vi "Application Example Advanced.vi"() -> ()   [LabVIEW 2015]
uses:
  <vilib>/Automotive Diagnostic Command Set/Diagnostic Protocols.llb/DTC Descriptor.ctl
  _SubVIs/DPID Periodic Rate.ctl
  _SubVIs/DPID Parameters.ctl
  <vilib>/Automotive Diagnostic Command Set/Diagnostic Protocols.llb/Diagnostic Trouble Code.ctl
  Engine/SubVIs/GMLAN/_SubVIs/DTCStatusMask.ctl
  <vilib>/Automotive Diagnostic Command Set/Diagnostic Transport.llb/Property ID.ctl
  <vilib>/xnet/xnet.llb/XNET Frame CAN.ctl
  <vilib>/xnet/xnet.llb/XNET Frame Type CAN.ctl
  _SubVIs/CAN Frame.ctl
  <vilib>/Automotive Diagnostic Command Set/Diagnostic Transport.llb/Transport Protocol Selector.ctl
  Engine/SubVIs/GMLAN/_SubVIs/ReadDataByPacketIdentifier_SubFunctions.ctl
  Engine/SubVIs/GMLAN/_SubVIs/DisableNormalCommunication_Parameter.ctl
  Engine/SubVIs/GMLAN/_SubVIs/ReadDiagnosticInformation_ByStatus.vi
  <vilib>/Utility/error.llb/Clear Errors.vi
  Engine/SubVIs/GMLAN/Utilities/GMLAN Service Broadcast.vi
  Engine/SubVIs/GMLAN/Utilities/Convert Raw Data to DTCs.vi
  <vilib>/xnet/xnet.llb/XNET Create Session (Frame Input Queued).vi
  <vilib>/Automotive Diagnostic Command Set/Diagnostic Transport.llb/Diagnostic Service.vi
  <vilib>/Automotive Diagnostic Command Set/Diagnostic Transport.llb/Apply Success Failure Error.vi
  <vilib>/Automotive Diagnostic Command Set/Diagnostic Transport.llb/Diag Globals.vi
  <vilib>/Automotive Diagnostic Command Set/Diagnostic Transport.llb/Diagnostic Service Send.vi
  <vilib>/Automotive Diagnostic Command Set/Diagnostic Transport.llb/Diagnostic Response Recv.vi
  <vilib>/Automotive Diagnostic Command Set/Diagnostic Transport.llb/Apply Diagnostic Error.vi
  <vilib>/xnet/xnet.llb/XNET Read (Frame CAN).vi
  <vilib>/Automotive Diagnostic Command Set/Diagnostic Protocols.llb/Convert to Phys.vi
  <vilib>/xnet/xnet.llb/XNET Database Close (Database).vi
  <vilib>/addons/Automotive Diagnostic Command Set/NI_Automotive Diagnostic Command Set.lvlib
  Engine/SubVIs/GMLAN/GMLAN.lvlib
panel:
  in  "Enable Comm":bool
  out "Success?":bool=TRUE
  in  "Read DID":bool
  in  "Read PIDs":bool
  in  "Stop DPIDs":bool
  in  "Start DPIDs":bool
  in  "DTC Reset":bool
  in  "Read DTCs":bool
  in  "Setup DPIDs":bool
  in  "Enable Comm":bool
  in  "Write CPID":bool
  in  "Disable Comm":bool
  in  "Tab Control":T1(tab)
  in  "HW select":u16(ring) items=["NI-XNET", "NI-CAN"]
  in  "CAN Interface":string(combo)="CAN1"
  in  "Baudrate":u32=500000
  in  "Receive ID":u32=2024 format="%.0x"
  in  "Transmit ID":u32=2016 format="%.0x"
  in  "UUDT Receive ID":u32=1512 format="%.0x"
  in  "DPIDs":T3(array[cluster])=[{"DPID ID"=239, "Speed"=enum."Medium", "PIDs"=[14]}, {"DPID ID"=253, "Speed"=enum."Fast", "PIDs"=[12]}] {"PIDs" format="%.0x"; "DPID ID" format="%.0x"}
  in  "DTC descriptor":T4={"DTC Byte Length"=2, "Status Byte Length"=1, "Add Data Byte Length"=1, "Byte Order"=enum."Motorola"}
  in  "DID ID":u8=153 format="%.0x"
  out "DID Data":u8[](array[numeric])=[32, 8, 18, 17]
  out "PID Data":u8[](array[numeric])=[128]
  in  "PID ID":u16=14 format="%.0x"
  in  "CPID ID":u8=29 format="%.0x"
  in  "CPIDControlBytes":u8[](array[numeric])=[0, 0, 0, 0, 0] format="%.0x"
  out "DPID":T5={"DPID ID"=253, "Speed"=enum."Fast", "PIDs"=[12]}
  out "timestamp":timestamp=timestamp(3432175878.295675 s since 1904-01-01)
  out "payload":u8[](array[numeric])
  out "EndofDTCReport":bool=TRUE
  out "DTCs":T6[](array[typedef])
  in  "status mask":T7={"DTC supported by calibration"=FALSE, "current DTC"=TRUE, "test not passed since DTC cleared"=FALSE, "test failed since DTC cleared"=FALSE, "history DTC"=FALSE, "test not passed since current power up"=FALSE, "current DTC since power up"=FALSE, "warning indicator requested state"=FALSE}
  out "error IO":errorcluster
  in  "stop":bool
  out "stopped?":bool=TRUE
  # "$90 - VehicleIdentificationNumber (VIN)\n$92\t- System Supplier ID\n$97\t- SystemNameOrEngineType"
  # "$C - Engine Speed\n$E\t- Spark Advance"
  # "x10 CDAR\nx1D PHSR"
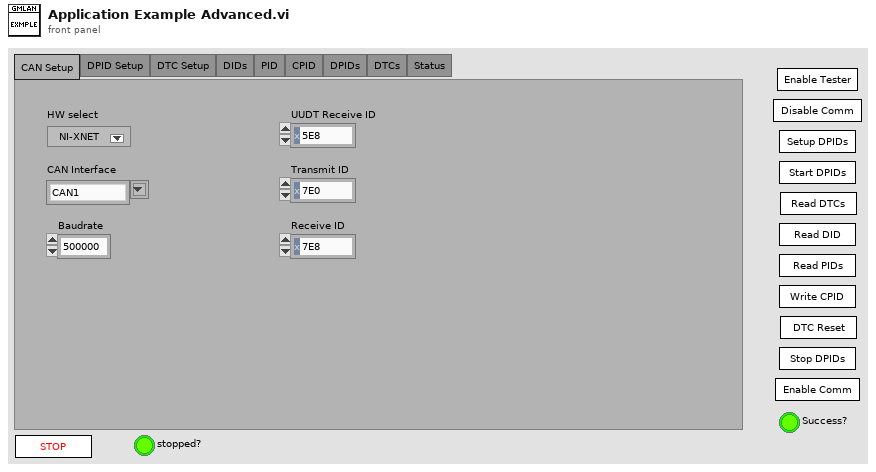
[diagram p1: front panel]
types:
  T1 = enum32{"CAN Setup", "DPID Setup", "DTC Setup", "DIDs", "PID", "CPID", "DPIDs", "DTCs", "Status"}
  T2 = typedef "DPID Periodic Rate.ctl" = enum16{"Slow", "Medium", "Fast"}
  T3 = cluster{"DPID ID":u8, "Speed":T2, "PIDs":u16[]}[]
  T4 = typedef "DTC Descriptor.ctl" = cluster{"DTC Byte Length":i32, "Status Byte Length":i32, "Add Data Byte Length":i32, "Byte Order":enum16{"Motorola", "Intel"}}
  T5 = typedef "DPID Parameters.ctl" = cluster{"DPID ID":u8, "Speed":T2, "PIDs":u16[]}
  T6 = typedef "Diagnostic Trouble Code.ctl" = cluster{"DTC":u32, "Status":u32, "Add Data":u32}
  T7 = typedef "GMLAN.lvlib/DTCStatusMask.ctl" = cluster{"DTC supported by calibration":bool, "current DTC":bool, "test not passed since DTC cleared":bool, "test failed since DTC cleared":bool, "history DTC":bool, "test not passed since current power up":bool, "current DTC since power up":bool, "warning indicator requested state":bool}
  T8 = typedef "CAN Frame.ctl" = cluster{"Frame name":string, "Identifier":u32, "Payload Length":u32, "Timing Type":u32, "Transmit Time":dbl, "Extended Identifier?":bool, "Comment":string}
  T9 = typedef "XNET Frame CAN.ctl" = cluster{"timestamp":timestamp, "payload":u8[], "identifier":u32, "type":T10, "extended?":bool, "echo?":bool}
  T10 = typedef "XNET Frame Type CAN.ctl" = u8
  T11 = typedef "NI_Automotive Diagnostic Command Set.lvlib/Property ID.ctl" = enum16{"Timeout Diag Command", "Timeout FC (Bs)", "Timeout CF (Cr)", "Receive Block Size (BS)", "Wait Time CF (STmin)", "Max Wait Frames (N_WFTmax)", "Wait Frames to Send (N_WAIT)", "Time between Waits (T_W)", "Fill CAN Frames", "Fill Byte", "Invalid Response as Error", "Max RspPending Count", "VWTP Command Timeout", "STmin", "P2min", "Termination"}
  T12 = typedef "NI_Automotive Diagnostic Command Set.lvlib/Transport Protocol Selector.ctl" = enum16{"ISO TP - Normal Mode", "ISO TP - Mixed Mode", "VW TP 2.0", "Diagnostics on IP", "ISO TP LIN"}
  T13 = typedef "NI_Automotive Diagnostic Command Set.lvlib/Diag Reference.ctl" = cluster{"Diag CAN Handle":u32, "Transport Protocol":T12, "Receive Address Extension":u8, "Transmit Address Extension":u8, "Receive CAN Id":u32, "Transmit CAN Id":u32, "Diag CAN Queue":refnum<queue>, "Log Frames ?":bool, "My TP Address":u8, "Other TP Address":u8, "T1":u16, "T2":u16, "T3":u16, "T4":u16, "Tx SN":u8, "Block Size":u8, "Rx SN":u8, "VW TP Initialized?":bool, "Tx block no":u8, "baud rate":u32, "Interface":string, "Channel Diag CAN Handle":u32, "UDP Connection ID":refnum<k16>, "TCP Connection ID":refnum<k5>, "Target IP Addr":u32, "Source Address":u16, "Target Address":u16, "Send Header NACK?":bool, "DLL Handle":u32, "NAD":u8, "Time Stamp read first":dbl, "Time Stamp read last":dbl, "Time Stamp write first":dbl, "Time Stamp write last":dbl, "Time Stamp write":dbl, "Time Stamp read":dbl}
  T14 = enum8{"Idle", "Read DID", "Read DTCs", "Reset DTCs", "Setup DPIDs", "Start DPIDs", "Stop DPIDs", "Read PID", "Write CPID", "DisableCommunication", "EnableCommunication", "Stop"}
  T15 = typedef "GMLAN.lvlib/ReadDataByPacketIdentifier_SubFunctions.ctl" = enum8{"stopSending", "sendOneResponse", "scheduleAtSlowRate", "scheduleAtMediumRate", "scheduleAtFastRate"}
  T16 = typedef "GMLAN.lvlib/DisableNormalCommunication_Parameter.ctl" = enum8{"SpecificECU", "EntireNetwork"}
  T17 = typedef "Filtered DPID IDs.ctl" = cluster{"Slow":u8[], "Medium":u8[], "Fast":u8[]}
  T18 = typedef "NI_Automotive Diagnostic Command Set.lvlib/Diag CAN Frame Log.ctl" = cluster{"Timestamp":dbl, "ArbitrationId":u32, "IsRemote":u8, "DataLength":u8, "Data":u8[]}
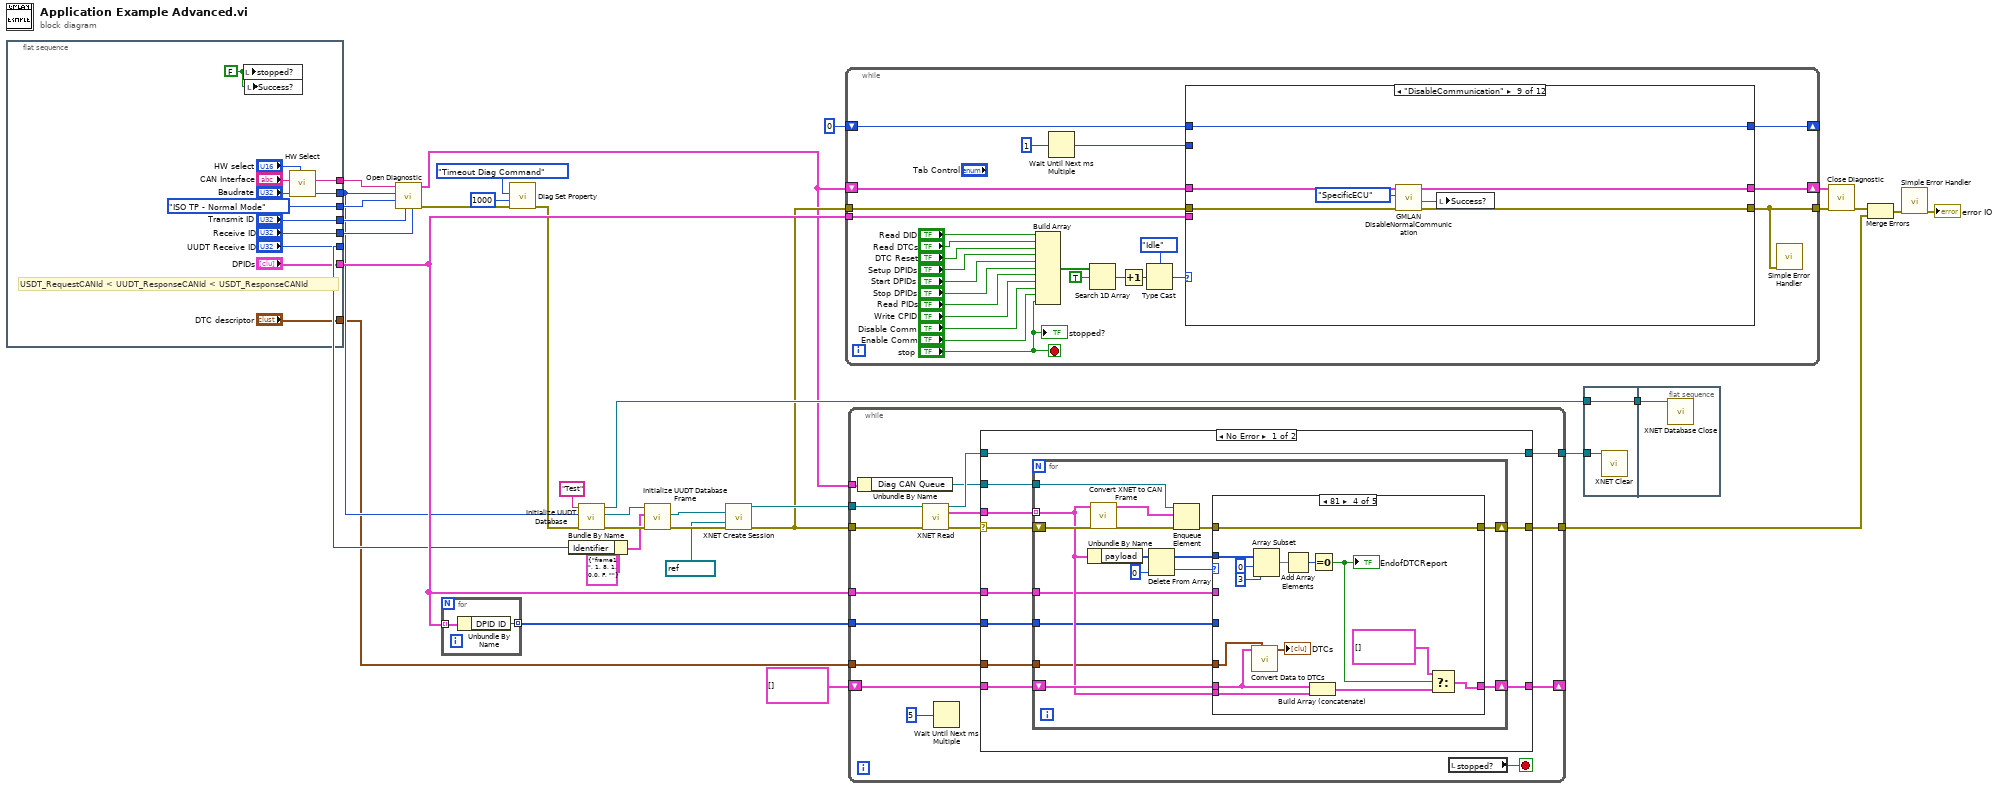
[diagram p0: block diagram]
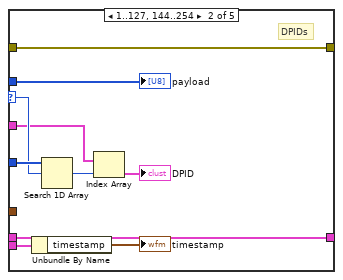
[diagram p3: hidden frame]
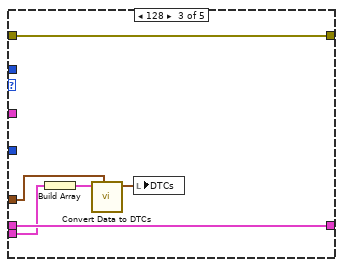
[diagram p4: hidden frame]
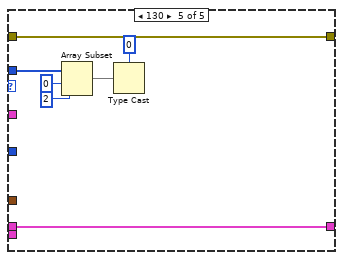
[diagram p5: hidden frame]
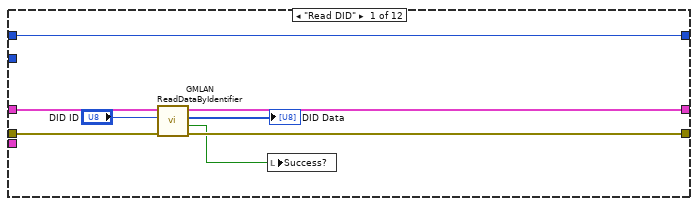
[diagram p7: hidden frame]
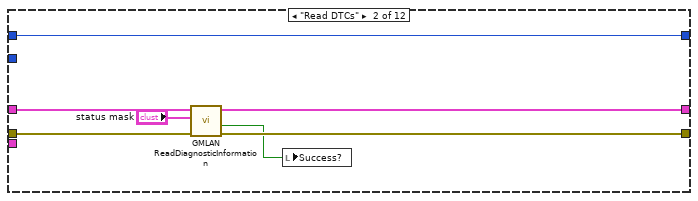
[diagram p8: hidden frame]
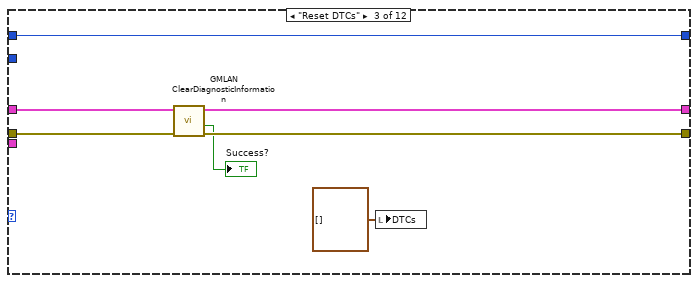
[diagram p9: hidden frame]
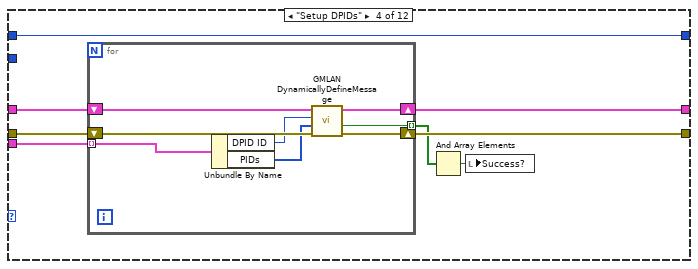
[diagram p10: hidden frame]
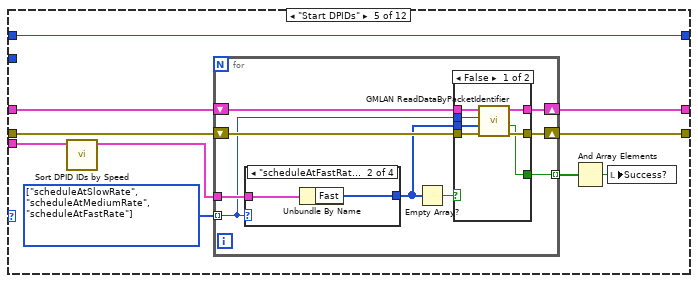
[diagram p11: hidden frame]
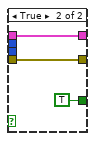
[diagram p12: hidden frame]
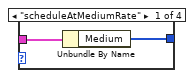
[diagram p13: hidden frame]
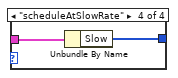
[diagram p15: hidden frame]
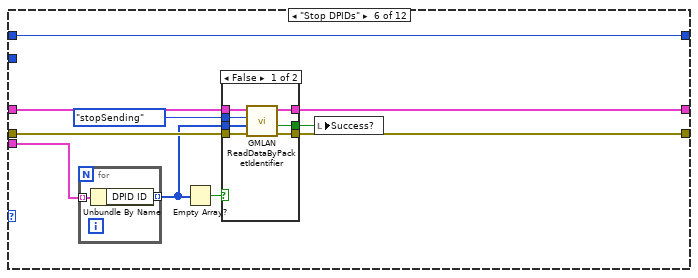
[diagram p16: hidden frame]
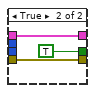
[diagram p17: hidden frame]
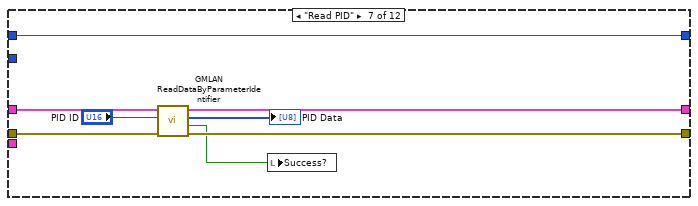
[diagram p18: hidden frame]
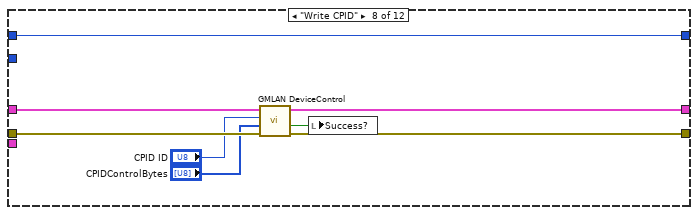
[diagram p19: hidden frame]
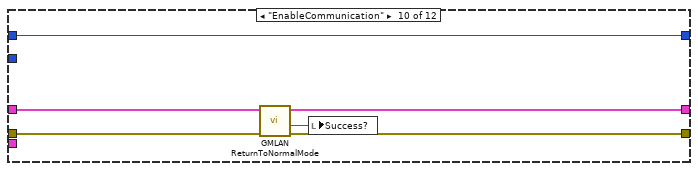
[diagram p20: hidden frame]
diagram:
  n1 = flat-sequence {
    tunnel: [w46] -> w33
    tunnel: ["Baudrate"] -> w2
    tunnel: [Transport_Protocol_Selector."ISO TP - Normal Mode" ("Transport Protocol")] -> w32
    tunnel: ["Transmit ID"] -> w31
    tunnel: ["Receive ID"] -> w30
    tunnel: ["UUDT Receive ID"] -> w11
    tunnel: ["DTC descriptor"] -> w1
    tunnel: ["DPIDs"] -> w20
    frame #0 {
      w36 = FALSE ("stopped?")
      # "USDT_RequestCANId < UUDT_ResponseCANId < USDT_ResponseCANId"
      n2 = local write "stopped?"(w36) -> ()
      n3 = local write "Success?"(w36) -> ()
      n4 = call "HW Select.vi"("HW select"="HW select", "CAN port"="CAN Interface") -> ("CAN port out"=w46:string)  [unwired: 9 in]
    }
  }
  n5 = call <vilib>:"Open Diagnostic.vi"("Receive ID"=w30, "Transmit ID"=w31, "Transport Protocol"=w32, "Baud Rate"=w2, "CAN Interface"=w33) -> ("error out"=w29:errorcluster, "diag ref out"=w4:T13)  [unwired: 1 in, 4 out]
  n6 = for {
    tunnel: w20 -> [w48] mode=indexing
    tunnel: [w47] -> w26 mode=indexing
    n7 = Unbundle By Name(w48) -> ("DPID ID"=w47:u8)
  }
  n8 = call <vilib>:"Diag Set Property.vi"("error in (no error)"=w29, "property value"=u32 1000, "property ID"=Property_ID."Timeout Diag Command") -> ("error out"=w6:errorcluster)  [unwired: 7 in, 1 out]
  n9 = Bundle By Name(cluster=T8 {"Frame name"="frame1", "Identifier"=1, "Payload Length"=8, "Timing Type"=1, "Transmit Time"=0.0, "Extended Identifier?"=FALSE, "Comment"=""} ("CAN Frame"), "Identifier"=w11) -> (w9:T8)
  n10 = call "Initialize UUDT Database.vi"("error in (no error)"=w6, "Baud Rate"=w2, "Addon Name"="Test") -> ("error out"=w16:errorcluster, "Cluster"=w15:refnum<k21>, "XNET Database"=w7:refnum<k21>)  [unwired: 6 in]
  n11 = call "Initialize UUDT Database Frame.vi"("error in"=w16, "CAN Frame"=w9, "cluster in"=w15) -> ("error out"=w13:errorcluster, "frame out"=w14:refnum<k21>)  [unwired: 6 in, 1 out]
  n12 = call-poly <vilib>:"XNET Create Session.vi"("frame"=w14, "interface"=refnum<k21> "CAN1", "error in (no error)"=w13) -> ("session out"=w17:refnum<k21>, "error out"=w5:errorcluster)  [unwired: 11 out]
  n13 = while {
    tunnel: w5 -> [w73]
    tunnel: [w52] -> w34
    shift-right: [w72] -> w35
    shift-left: w4 -> [w74]
    shift-right: [w66] -> _
    shift-left: u32 0 ("millisecond timer value") -> [w64]
    tunnel: w20 -> [w60]
    stop <- "stop" stop-if-true
    n14 = Build Array("Read DID", "Read DTCs", "DTC Reset", "Setup DPIDs", "Start DPIDs", "Stop DPIDs", "Read PIDs", "Write CPID", "Disable Comm", "Enable Comm", "stop") -> (w70:bool[])
    n15 = Wait Until Next ms Multiple(millisecond multiple=1) -> (millisecond timer value=w65:u32)
    n16 = Search 1D Array(1D array=w70, element=TRUE) -> (index of element=w57:i32)  [unwired: 1 in]
    n17 = Increment(x=w57) -> (x+1=w55:u8)
    n18 = Type Cast(type=T14."Idle", x=w55) -> (*(type *) &x=w54:T14)
    n19 = case shown="\"DisableCommunication\"" w54 {
      tunnel: w74 -> [w82 w88 w96 w101 w120 w155 w177 w184 w191 w197 w199 w212]
      tunnel: w73 -> [w81 w86 w95 w103 w122 w157 w176 w185 w192 w198 w200 w213]
      tunnel: [w80 w84 w94 w100 w119 w154 w175 w182 w189 w195 w199 w210] -> w72
      tunnel: [w79 w85 w93 w102 w121 w156 w174 w183 w190 w196 w200 w211] -> w52
      tunnel: w65 -> [_ _ _ _ _ _ _ _ _ _ _ w208]
      tunnel: [w75 w89 w92 w104 w118 w153 w170 w181 w188 w194 w201 w209] -> w66
      tunnel: w64 -> [w75 w89 w92 w104 w118 w153 w170 w181 w188 w194 w201 w204]
      tunnel: w60 -> [_ _ _ w99 w117 w152 _ _ _ _ _ _]
      frame "Read DID" {
        n20 = call "GMLAN ReadDataByIdentifier.vi"("error in (no error)"=w81, "Data ID (DID)"="DID ID", "diag ref in"=w82) -> ("error out"=w79:errorcluster, "success?"=w78:bool, "data out"=→"DID Data":u8[], "diag ref out"=w80:T13)  [unwired: 5 in]
        n21 = local write "Success?"(w78) -> ()
      }
      frame "Read DTCs" {
        n22 = call-poly "GMLAN ReadDiagnosticInformation.vi"("error in (no error)"=w86, "status mask"="status mask", "diag ref in"=w88) -> ("error out"=w85:errorcluster, "success?"=w83:bool, "diag ref out"=w84:T13)  [unwired: 5 in, 1 out]
        n23 = local write "Success?"(w83) -> ()
      }
      frame "Reset DTCs" {
        n24 = call "GMLAN ClearDiagnosticInformation.vi"("error in (no error)"=w95, "diag ref in"=w96) -> ("error out"=w93:errorcluster, "success?"=→"Success?":bool, "diag ref out"=w94:T13)  [unwired: 7 in]
        n25 = local write "DTCs"(T6[] [] ("DTCs")) -> ()
      }
      frame "Setup DPIDs" {
        n26 = for {
          shift-right: [w111] -> w102
          shift-left: w103 -> [w112]
          shift-right: [w109] -> w100
          shift-left: w101 -> [w110]
          tunnel: w99 -> [w108] mode=indexing
          tunnel: [w105] -> w98 mode=indexing
          n27 = Unbundle By Name(w108) -> ("DPID ID"=w107:u8, "PIDs"=w106:u16[])
          n28 = call "GMLAN DynamicallyDefineMessage.vi"("error in (no error)"=w112, "PID List"=w106, "DPID ID"=w107, "diag ref in"=w110) -> ("error out"=w111:errorcluster, "success?"=w105:bool, "diag ref out"=w109:T13)  [unwired: 5 in]
        }
        n29 = And Array Elements(Boolean array=w98) -> (logical AND=w97:bool)
        n30 = local write "Success?"(w97) -> ()
      }
      frame "Start DPIDs" {
        w115 = T15[] [enum."scheduleAtSlowRate", enum."scheduleAtMediumRate", enum."scheduleAtFastRate"] items=["stopSending", "sendOneResponse", "scheduleAtSlowRate", "scheduleAtMediumRate", "scheduleAtFastRate"]
        n31 = call "Sort DPID IDs by Speed.vi"("DPIDs"=w117) -> ("Filtered DPIDs IDs"=w116:T17)  [unwired: 10 in]
        n32 = for {
          tunnel: w116 -> [w127]
          shift-right: [w130] -> w121
          shift-left: w122 -> [w131]
          shift-right: [w128] -> w119
          shift-left: w120 -> [w129]
          tunnel: w115 -> [w124] mode=indexing
          tunnel: [w123] -> w113 mode=indexing
          n33 = case shown="\"scheduleAtFastRate\"" w124 {
            tunnel: w127 -> [w143 w145 _ w147]
            tunnel: [w142 w144 _ w146] -> w126
            frame "scheduleAtMediumRate" {
              n34 = Unbundle By Name(w143) -> ("Medium"=w142:u8[])
            }
            frame "scheduleAtFastRate" {
              n35 = Unbundle By Name(w145) -> ("Fast"=w144:u8[])
            }
            frame Default {
            }
            frame "scheduleAtSlowRate" {
              n36 = Unbundle By Name(w147) -> ("Slow"=w146:u8[])
            }
          }
          n37 = Empty Array?(array=w126) -> (empty?=w125:bool)
          n38 = case shown="False" w125 {
            tunnel: w131 -> [w138 w140]
            tunnel: [w137 w140] -> w130
            tunnel: w129 -> [w136 w141]
            tunnel: [w135 w141] -> w128
            tunnel: w124 -> [w134 _]
            tunnel: w126 -> [w133 _]
            tunnel: [w132 TRUE ("success?")] -> w123
            frame False {
              n39 = call "GMLAN ReadDataByPacketIdentifier.vi"("error in (no error)"=w138, "DPIDs"=w133, "Sub Function"=w134, "diag ref in"=w136) -> ("error out"=w137:errorcluster, "success?"=w132:bool, "diag ref out"=w135:T13)  [unwired: 4 in, 1 out]
            }
            frame True {
            }
          }
        }
        n40 = And Array Elements(Boolean array=w113) -> (logical AND=w114:bool)
        n41 = local write "Success?"(w114) -> ()
      }
      frame "Stop DPIDs" {
        n42 = for {
          tunnel: w152 -> [w169] mode=indexing
          tunnel: [w168] -> w150 mode=indexing
          n43 = Unbundle By Name(w169) -> ("DPID ID"=w168:u8)
        }
        n44 = Empty Array?(array=w150) -> (empty?=w151:bool)
        n45 = case shown="False" w151 {
          tunnel: w157 -> [w164 w166]
          tunnel: [w163 w166] -> w156
          tunnel: w155 -> [w162 w167]
          tunnel: [w161 w167] -> w154
          tunnel: ReadDataByPacketIdentifier_SubFunctions."stopSending" ("Sub Function") -> [w160 _]
          tunnel: w150 -> [w159 _]
          tunnel: [w158 TRUE ("success?")] -> w148
          frame False {
            n46 = call "GMLAN ReadDataByPacketIdentifier.vi"("error in (no error)"=w164, "DPIDs"=w159, "Sub Function"=w160, "diag ref in"=w162) -> ("error out"=w163:errorcluster, "success?"=w158:bool, "diag ref out"=w161:T13)  [unwired: 4 in, 1 out]
          }
          frame True {
          }
        }
        n47 = local write "Success?"(w148) -> ()
      }
      frame "Read PID" {
        n48 = call "GMLAN ReadDataByParameterIdentifier.vi"("error in (no error)"=w176, "Parameter ID (PID)"="PID ID", "diag ref in"=w177) -> ("error out"=w174:errorcluster, "success?"=w173:bool, "data out"=→"PID Data":u8[], "diag ref out"=w175:T13)  [unwired: 5 in]
        n49 = local write "Success?"(w173) -> ()
      }
      frame "Write CPID" {
        n50 = call "GMLAN DeviceControl.vi"("error in (no error)"=w185, "CPIDControlBytes"="CPIDControlBytes", "CPID ID"="CPID ID", "diag ref in"=w184) -> ("error out"=w183:errorcluster, "success?"=w180:bool, "diag ref out"=w182:T13)  [unwired: 5 in]
        n51 = local write "Success?"(w180) -> ()
      }
      frame "DisableCommunication" {
        n52 = call "GMLAN DisableNormalCommunication.vi"("error in (no error)"=w192, "Parameter"=DisableNormalCommunication_Parameter."SpecificECU", "diag ref in"=w191) -> ("error out"=w190:errorcluster, "success?"=w186:bool, "diag ref out"=w189:T13)  [unwired: 6 in]
        n53 = local write "Success?"(w186) -> ()
      }
      frame "EnableCommunication" {
        n54 = call "GMLAN ReturnToNormalMode.vi"("error in (no error)"=w198, "diag ref in"=w197) -> ("error out"=w196:errorcluster, "success?"=w193:bool, "diag ref out"=w195:T13)  [unwired: 7 in]
        n55 = local write "Success?"(w193) -> ()
      }
      frame "Stop" {
      }
      frame Default {
        # "Tester Present"
        n56 = Subtract(x=w208, y=w204) -> (x-y=w207:u32)
        n57 = Greater Or Equal?(x=w207, y=u32 1000) -> (x >= y?=w205:bool)
        n58 = Compound Arithmetic op=AND(w205, "Enable Comm") -> (w203:bool)
        n59 = case shown="True" w203 {
          tunnel: w213 -> [w215 w221]
          tunnel: w212 -> [w216 w220]
          tunnel: [w215 w219] -> w211
          tunnel: [w216 w218] -> w210
          tunnel: w208 -> [_ w217]
          tunnel: [w214 w217] -> w209
          tunnel: w204 -> [w214 _]
          frame False {
          }
          frame True {
            n60 = call "GMLAN TesterPresent.vi"("error in (no error)"=w221, "diag ref in"=w220) -> ("error out"=w219:errorcluster, "diag ref out"=w218:T13)  [unwired: 7 in, 1 out]
          }
        }
      }
    }
    n61 = call <vilib>:"Simple Error Handler.vi"("error in (no error)"=w52) -> ()  [unwired: 4 in, 5 out]
    "stopped?" <- "stop"
  }
  n62 = while {
    tunnel: w5 -> [w234]
    shift-right: [w230] -> _
    shift-left: T9[] [] ("data") -> [w231]
    tunnel: w1 -> [w229]
    tunnel: [w227] -> w24
    tunnel: w20 -> [w226]
    tunnel: w26 -> [w225]
    tunnel: w17 -> [w235]
    tunnel: [w224] -> w18
    tunnel: w4 -> [w223]
    stop <- w237 stop-if-true
    n63 = Unbundle By Name(w223) -> ("Diag CAN Queue"=w222:refnum<queue>)
    n64 = call-poly <vilib>:"XNET Read.vi"("session in"=w235, "error in (no error)"=w234) -> ("session out"=w228:refnum<k21>, "data"=w232:T9[], "error out"=w233:errorcluster)  [unwired: 10 in, 1 out]
    n65 = Wait Until Next ms Multiple(millisecond multiple=5) -> ()  [unwired: 1 out]
    n66 = case shown="No Error" w233 {
      selector: w233 -> [w245 w304]
      tunnel: w232 -> [w238 _]
      tunnel: [w244 w304] -> w227
      tunnel: w231 -> [w247 w303]
      tunnel: [w246 w303] -> w230
      tunnel: w222 -> [w243 _]
      tunnel: w229 -> [w242 _]
      tunnel: w228 -> [w239 w302]
      tunnel: w226 -> [w241 _]
      tunnel: w225 -> [w240 _]
      tunnel: [w239 w302] -> w224
      frame No Error {
        n67 = for {
          tunnel: w238 -> [w254] mode=indexing
          shift-right: [w260] -> w246
          shift-left: w247 -> [w261]
          shift-right: [w259] -> w244
          shift-left: w245 -> [w258]
          tunnel: w243 -> [w256]
          tunnel: w242 -> [w252]
          tunnel: w241 -> [w251]
          tunnel: w240 -> [w250]
          n68 = Unbundle By Name(w254) -> ("payload"=w253:u8[])
          n69 = call "Convert XNET to CAN Frame.vi"("XNET frame"=w254) -> ("CAN Frame"=w255:T18)  [unwired: 10 in]
          n70 = Delete From Array(array=w253, index=0) -> (deleted portion=w262:u8, array with subset deleted=w248:u8[])  [unwired: 1 in]
          n71 = Enqueue Element(queue=w256, element=w255, error in (no error)=w258) -> (error out=w257:errorcluster)  [unwired: 1 in, 2 out]
          n72 = case shown="81" w262 {
            selector: w262 -> [_ w272 _ _ _]
            tunnel: w248 -> [_ w265 _ w294 w297]
            tunnel: w261 -> [w264 w274 w280 w281 w301]
            tunnel: w254 -> [_ w268 w278 w288 _]
            tunnel: [w264 w274 w280 w286 w301] -> w260
            tunnel: [w263 w266 w279 w285 w300] -> w259
            tunnel: w257 -> [w263 w266 w279 w285 w300]
            tunnel: w252 -> [_ _ w276 w283 _]
            tunnel: w251 -> [_ w270 _ _ _]
            tunnel: w250 -> [_ w273 _ _ _]
            frame Default {
            }
            frame 1..127, 144..254 {
              # "DPIDs"
              n73 = Unbundle By Name(w268) -> ("timestamp"=→"timestamp":timestamp)
              n74 = Search 1D Array(1D array=w273, element=w272) -> (index of element=w271:i32)  [unwired: 1 in]
              n75 = Index Array(array=w270, index=w271) -> (element=→"DPID":cluster{"DPID ID":u8, "Speed":T2, "PIDs":u16[]})
              "payload" <- w265
            }
            frame 128 {
              n76 = Build Array(w278) -> (w277:T9[])
              n77 = call "Convert Data to DTCs.vi"("DTC descriptor"=w276, "All DTCs"=w277) -> ("DTCs"=w275:T6[])  [unwired: 8 in, 1 out]
              n78 = local write "DTCs"(w275) -> ()
            }
            frame 129 {
              n79 = call "Convert Data to DTCs.vi"("DTC descriptor"=w283, "All DTCs"=w281) -> ("DTCs"=→"DTCs":T6[])  [unwired: 8 in, 1 out]
              n80 = Array Subset(array=w294, index=0, length=3) -> (w291:u8[])
              n81 = Add Array Elements(numeric array=w291) -> (sum=w290:u8)
              n82 = Build Array (concatenate)(w281, w288) -> (w284:T9[])
              n83 = Equal To 0?(x=w290) -> (x = 0?=w289:bool)
              "EndofDTCReport" <- w289
              n84 = Select(t=T9[] [] ("data"), s=w289, f=w284) -> (s? t:f=w286:T9[])
            }
            frame 130 {
              n85 = Array Subset(array=w297, index=0, length=2) -> (w296:u8[])
              n86 = Type Cast(type=u16 0 ("length"), x=w296) -> ()  [unwired: 1 out]
            }
          }
        }
      }
      frame Error {
      }
    }
    n87 = local read "stopped?"() -> (w237:bool)
  }
  n88 = flat-sequence {
    tunnel: w18 -> [w306]
    tunnel: [w305] -> w8
    tunnel: w7 -> [w305]
    tunnel: w8 -> [w307]
    frame #0 {
      n89 = call <vilib>:"XNET Clear.vi"("session in"=w306) -> ()  [unwired: 14 in, 1 out]
    }
    frame #1 {
      n90 = call-poly <vilib>:"XNET Database Close.vi"("database in"=w307) -> ()  [unwired: 14 in, 1 out]
    }
  }
  n91 = call <vilib>:"Close Diagnostic.vi"("error in (no error)"=w34, "diag ref in"=w35) -> ("error out"=w25:errorcluster)  [unwired: 9 out]
  n92 = Merge Errors(w25, w24) -> (w23:errorcluster)
  n93 = call <vilib>:"Simple Error Handler.vi"("error in (no error)"=w23) -> ("error out"=→"error IO":errorcluster)  [unwired: 1 in, 7 out]
